vi "getVersion.vi"(11 "ComPort":refnum<visa-resource-name>="COM10") -> (0 "error out":errorcluster, 3 "received":string)   [LabVIEW 2018]
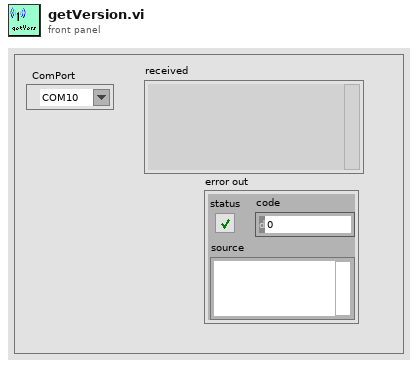
[diagram p1: front panel]
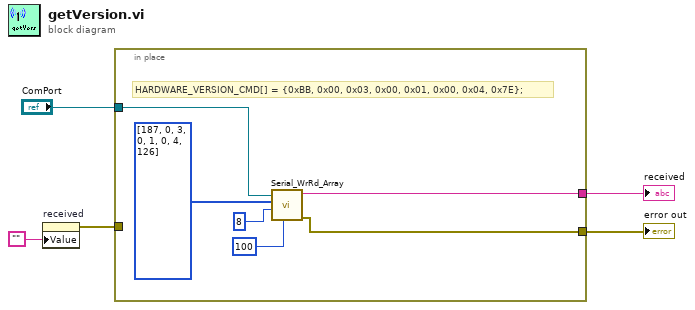
[diagram p0: block diagram]
diagram:
  n1 = property on="received" class="Str"("Value"="") -> (error out=w1:errorcluster)  [unwired: 2 in, 1 out]
  n2 = in-place {
    in-place-border: "ComPort" -> [w10]
    in-place-border: [w8] -> w4
    in-place-border: [w6] -> w3
    in-place-border: w1 -> [_]
    # "HARDWARE_VERSION_CMD[] = {0xBB, 0x00, 0x03, 0x00, 0x01, 0x00, 0x04, 0x7E};"
    n3 = call "Serial_WrRd_Array.vi"("Read Delay (ms)"=u16 100, "WR Size"=u16 8, "Array"=u8[] [187, 0, 3, 0, 1, 0, 4, 126], "ComPort"=w10) -> ("error out"=w6:errorcluster, "received"=w8:string)  [unwired: 5 in, 1 out]
  }
  "received" <- w4
  "error out" <- w3
